vi "scan frame to tip.vi"   [LabVIEW 2021]
uses:
  <userlib>/Nanonis Prog Interface V5/Nanonis Prog Interface.lvlib
panel:
  # "to Tip"
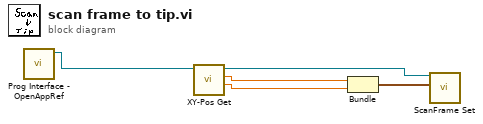
[diagram p0: block diagram]
diagram:
  n1 = call <userlib>:"Prog Interface - OpenAppRef.vi"() -> ("Application reference"=w4:refnum<vi>)  [unwired: 6 in, 1 out]
  n2 = call <userlib>:"XY-Pos Get.vi"("Application ref in"=w4) -> ("Y (m)"=w2:sgl, "X (m)"=w1:sgl, "Application ref out"=w5:refnum<vi>)  [unwired: 6 in, 1 out]
  n3 = Bundle("X (m)"=w1, "Y (m)"=w2) -> (w3:cluster{"X (m)":sgl, "Y (m)":sgl})  [unwired: 1 in]
  n4 = call <userlib>:"ScanFrame Set.vi"("Application ref in"=w5, "Center coordinates (m)"=w3) -> ()  [unwired: 12 in, 2 out]
